vi "Walk n laps.vi"   [LabVIEW 2016, in "ENED1120.lvrbt"]
uses:
  ENED1120.lvrbt
  <vilib>/NXT/NXTIO Xnodes/NXTIONodeSubVIs/NXTMotorRunDistance.vi
  <vilib>/NXT/Subs/LVHSConnector.ctl
  <vilib>/NXT/NXTIO Xnodes/AddressXNode/NXTIOAddress.xnode
  <vilib>/NXT/Block Support/NXT_OutputPort.ctl
  <vilib>/NXT/NXTIO Xnodes/NXTIOXNode/NXTIO.xnode
  <vilib>/NXT/LegoClasses/BrickReference/BrickReference.lvclass
types:
  T1 = typedef "NXT_OutputPort.ctl" = u8
  T2 = typedef "LVHSConnector.ctl" = refnum<class "BrickReference.lvclass">
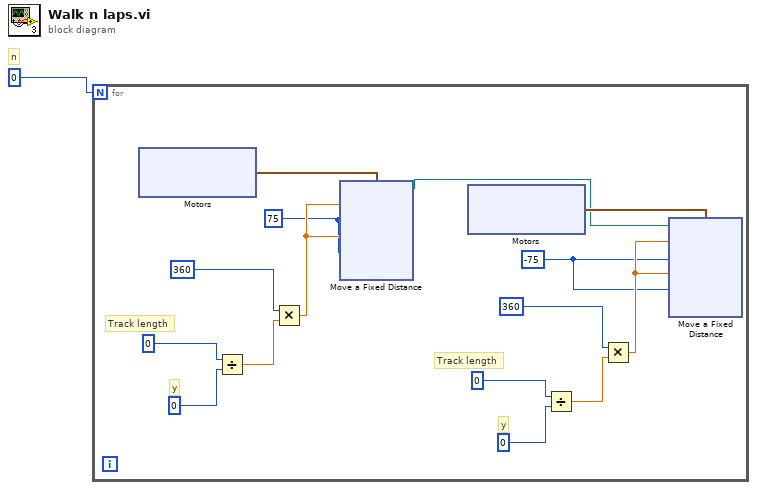
[diagram p0: block diagram]
diagram:
  # "n"
  n1 = for {
    N: 0 -> [_]
    w2 = i8 75 ("Speed 1")
    w4 = i8 -75 ("Speed 1")
    # "y"
    # "Track length"
    # "y"
    # "Track length"
    n2 = xnode "Motors"() -> ("Motor"=w16:cluster{"Port":T1, "Port":T1})
    n3 = Divide(x=0, y=0) -> (x/y=w12:dbl)
    n4 = Multiply(x=360 ("Distance 2"), y=w12) -> (x*y=w11:dbl)
    n5 = xnode "Move a Fixed Distance"("Speed 2"=w2, "Speed 1"=w2, "Distance 2"=w11, "Distance 1"=w11, "Motors"=w16) -> ("NXT/EV3"=w3:T2)  [unwired: 1 in]
    n6 = xnode "Motors"() -> ("Motor"=w10:cluster{"Port":T1, "Port":T1})
    n7 = Divide(x=0, y=0) -> (x/y=w6:dbl)
    n8 = Multiply(x=360 ("Distance 2"), y=w6) -> (x*y=w5:dbl)
    n9 = xnode "Move a Fixed Distance"("Speed 2"=w4, "Speed 1"=w4, "Distance 2"=w5, "Distance 1"=w5, "Motors"=w10, "NXT/EV3"=w3) -> ()  [unwired: 1 out]
  }
